vi "Check file and delete by byte.vi"(8 "error in (no error)":errorcluster, 10 "Delete if less than byte":i64=128, 11 "File in":refnum<file>) -> (0 "error out":errorcluster, 3 "deleted path out":path)   [LabVIEW 2020]
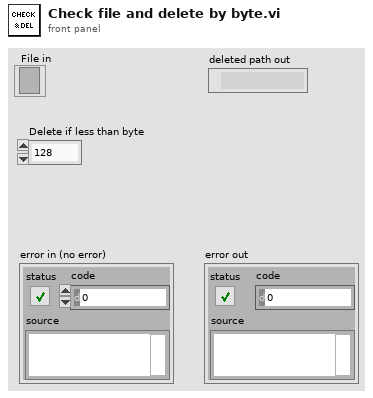
[diagram p1: front panel]
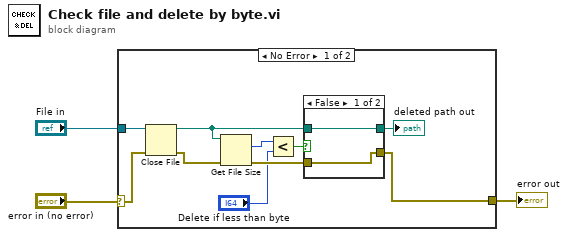
[diagram p0: block diagram]
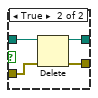
[diagram p2: hidden frame]
diagram:
  n1 = case shown="No Error" "error in (no error)" {
    selector: "error in (no error)" -> [w6 w20]
    tunnel: "File in" -> [w7 _]
    tunnel: [w5 w20] -> w1
    frame No Error {
      n2 = Close File(refnum=w7, error in=w6) -> (path=w10:path, error out=w12:errorcluster)
      n3 = Get File Size(file=w10, error in=w12) -> (size (in bytes)=w8:i64, 0:w13:errorcluster)  [unwired: 1 out]
      n4 = Less?(x=w8, y="Delete if less than byte") -> (x < y?=w11:bool)
      n5 = case shown="False" w11 {
        tunnel: w10 -> [w14 w19]
        tunnel: w13 -> [w15 w18]
        tunnel: [w15 w17] -> w5
        tunnel: [w14 w16] -> w4
        frame False {
        }
        frame True {
          n6 = Delete(path (use dialog)=w19, error in=w18) -> (deleted path=w16:path, error out=w17:errorcluster)  [unwired: 3 in, 1 out]
        }
      }
      "deleted path out" <- w4
    }
    frame Error {
    }
  }
  "error out" <- w1
